vi "Write background.vi"(8 "error in (no error)":errorcluster, 10 "background":dbl[](array[numeric]), 11 "Stresing_dual_cam in":refnum<class "Stresing_dual_cam.lvclass">) -> (0 "error out":errorcluster, 3 "Stresing_dual_cam out":refnum<class "Stresing_dual_cam.lvclass">)   [LabVIEW 2019, in "Stresing_dual_cam.lvclass"]
uses:
  Stresing_dual_cam.lvclass
  _cameraBase/_cameraBase.lvclass
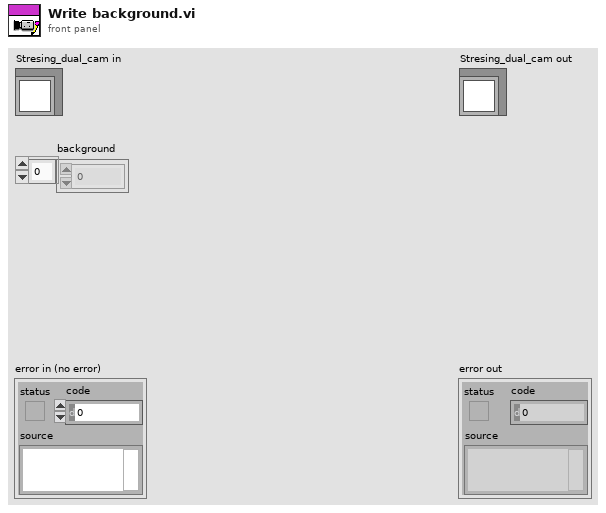
[diagram p1: front panel]
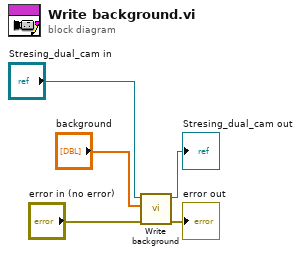
[diagram p0: block diagram]
diagram:
  n1 = call-parent "Write background.vi"("error in (no error)"="error in (no error)", "background"="background", "_cameraBase in"="Stresing_dual_cam in") -> ("error out"=→"error out":errorcluster, "_cameraBase out"=→"Stresing_dual_cam out":refnum<class "Stresing_dual_cam.lvclass">)  [unwired: 7 in]
